vi "mini_AC_test.vi"() -> ()   [LabVIEW 2016]
uses:
  <vilib>/Instr/_visa.llb/VISA Configure Serial Port (Instr).vi
panel:
  out "Waveform Chart":u8[](graph)
  out "return count":u32
  out "read buffer":string
  in  "write buffer":string="GAC,"
  in  "Serial Settings:Baud Rate":u32=9600
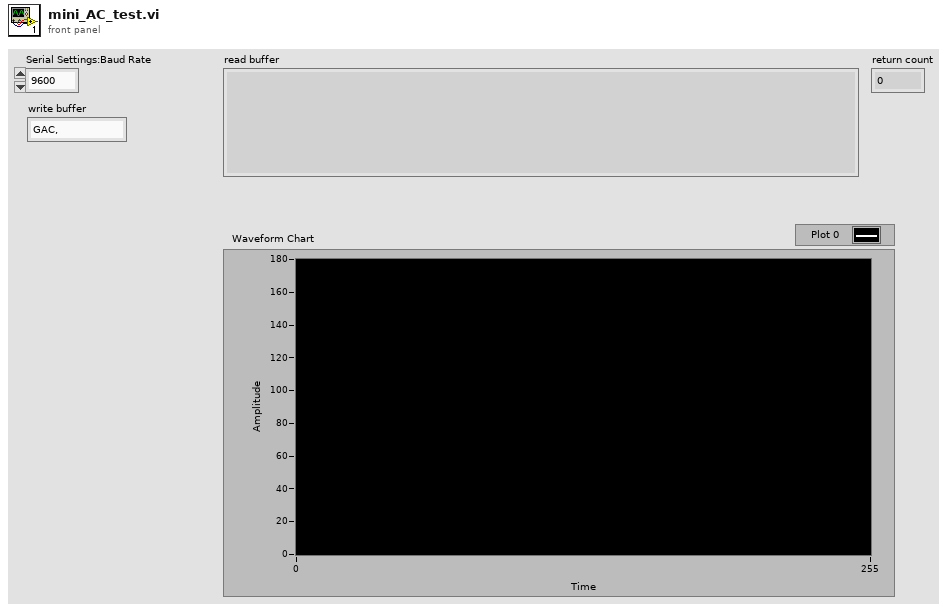
[diagram p1: front panel]
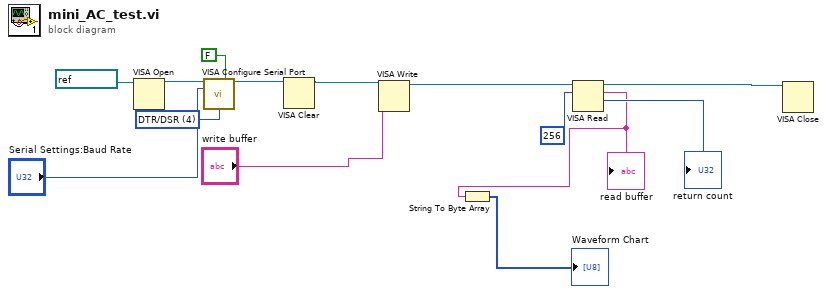
[diagram p0: block diagram]
diagram:
  w10 = u16 4 items=["None", "XON/XOFF", "RTS/CTS", "XON/XOFF & RTS/CTS", "DTR/DSR", "XON/XOFF & DTR/DSR"] ("flow control (0:none)")
  n1 = VISA Open(VISA resource name=refnum<visa-resource-name> "COM8") -> (VISA resource name=w12:refnum<visa-resource-name>)  [unwired: 4 in, 1 out]
  n2 = call-poly "VISA Configure Serial Port"("VISA resource name"=w12, "Enable Termination\nChar (T)"=FALSE ("Enable Termination\nChar (T)"), "baud rate (9600)"="Serial Settings:Baud Rate", "flow control (0:none)"=w10) -> ("VISA resource name out"=w8:refnum<visa-resource-name>)  [unwired: 10 in, 1 out]
  n3 = VISA Clear(VISA resource name=w8) -> (VISA resource name out=w7:refnum<visa-resource-name>)  [unwired: 1 in, 1 out]
  n4 = VISA Write(VISA resource name=w7, write buffer="write buffer") -> (VISA resource name out=w13:refnum<visa-resource-name>)  [unwired: 1 in, 2 out]
  n5 = VISA Read(VISA resource name=w13, byte count=u32 256) -> (VISA resource name out=w3:refnum<visa-resource-name>, read buffer=w2:string, return count=→"return count":u32)  [unwired: 1 in, 1 out]
  "read buffer" <- w2
  n6 = String To Byte Array(string=w2) -> (unsigned byte array=→"Waveform Chart":u8[])
  n7 = VISA Close(VISA resource name=w3) -> ()  [unwired: 1 in, 1 out]
